vi "Reg Get Bead Position.vi"(9 "Edge size":i32=12, 10 "Pixel Size (µm)":dbl, 11 "Image Ref":T1) -> (2 "Y Pos":dbl, 3 "X Pos":dbl)   [LabVIEW 2016]
uses:
  <vilib>/vision/Image Controls.llb/IMAQ Image.ctl
  Display Module/Display Module Custom Controls/ROI Descriptor.ctl
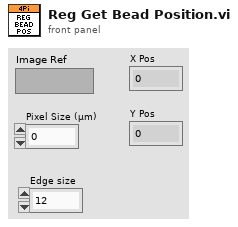
[diagram p1: front panel]
types:
  T1 = typedef "IMAQ Image.ctl" = refnum<image>
  T2 = typedef "ROI Descriptor.ctl" = cluster{"Global Rectangle":i32[], "Contours":cluster{"Contour Type":u32, "ROI Type":u32, "Points":i32[]}[]}
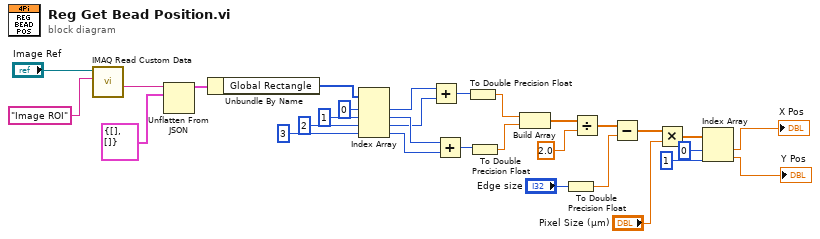
[diagram p0: block diagram]
diagram:
  n1 = call "IMAQ Read Custom Data"("Key"="Image ROI", "Image"="Image Ref") -> ("Custom Data Out"=w5:string)  [unwired: 7 in, 2 out]
  n2 = Unflatten From JSON(JSON string=w5, type and defaults=T2 {"Global Rectangle"=[], "Contours"=[]} ("Image ROI Descriptor")) -> (value=w7:T2)  [unwired: 5 in, 1 out]
  n3 = Unbundle By Name(w7) -> ("Global Rectangle"=w12:i32[])
  n4 = Index Array(array=w12, index #1=0 ("index"), index #2=1 ("index"), index #3=2 ("index"), index #4=3 ("index")) -> (element #1=w13:i32, element #2=w15:i32, element #3=w14:i32, element #4=w16:i32)
  n5 = Add(x=w13, y=w14) -> (x+y=w17:i32)
  n6 = Add(x=w15, y=w16) -> (x+y=w18:i32)
  n7 = To Double Precision Float(number=w17) -> (double precision float=w23:dbl)
  n8 = To Double Precision Float(number=w18) -> (double precision float=w24:dbl)
  n9 = Build Array(w23, w24) -> (w25:dbl[])
  n10 = To Double Precision Float(number="Edge size") -> (double precision float=w1:dbl)
  n11 = Divide(x=w25, y=2.0) -> (x/y=w21:dbl[])
  n12 = Subtract(x=w21, y=w1) -> (x-y=w22:dbl[])
  n13 = Multiply(x=w22, y="Pixel Size (µm)") -> (x*y=w26:dbl[])
  n14 = Index Array(array=w26, index #1=0 ("index"), index #2=1 ("index")) -> (element #1=→"X Pos":dbl, element #2=→"Y Pos":dbl)
